vi "Test Runner Error Codes.vi"(8 "error in (no error)":errorcluster) -> (0 "error out":errorcluster)   [LabVIEW 2013]
uses:
  classes/Test Runner.Folder/Test Runner.Folder.lvclass
  classes/Test Runner/Test Runner.lvclass/Test Runner.ctl
  classes/Assert/Assert Equal Value_Variant.vi
  classes/Test/Test.lvclass
  classes/Assert/Assert.lvclass
  classes/Test Runner/Test Runner.lvclass
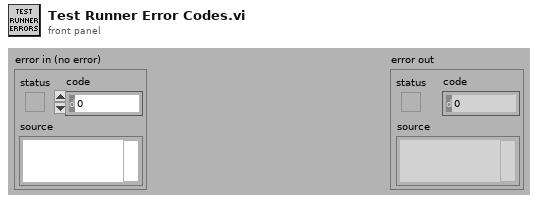
[diagram p1: front panel]
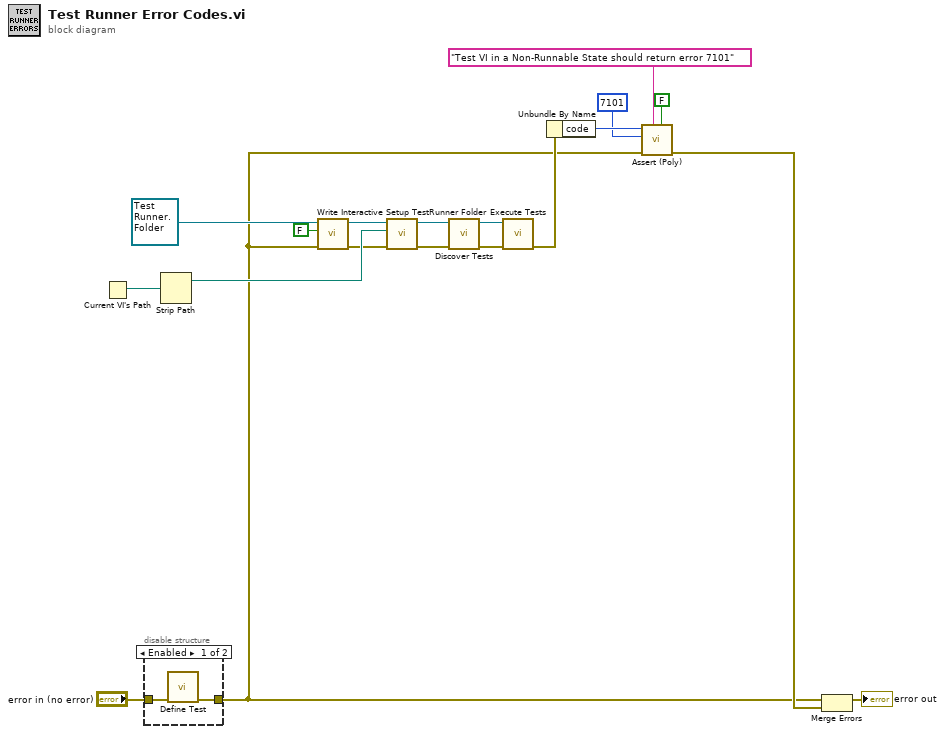
[diagram p0: block diagram]
diagram:
  n1 = Current VI's Path() -> (path=w7:path)
  n2 = disable-structure shown="Enabled" {
    disable-tunnel: "error in (no error)" -> [w20 w21]
    disable-tunnel: [w19 w21] -> w1
    frame Enabled {
      n3 = call "Define Test.vi"("error in (no error)"=w20) -> ("error out"=w19:errorcluster)  [unwired: 10 in]
    }
    frame Disabled {
    }
  }
  n4 = Strip Path(path=w7) -> (stripped path=w6:path)  [unwired: 1 out]
  n5 = call "Write Interactive.vi"("Interactive"=FALSE, "Test Runner in"=refnum<class "Test Runner.Folder.lvclass"> refnum ("Caraya.lvlib:Test Runner.Folder.lvclass")) -> ("Test Runner out"=w5:refnum<class "Test Runner.Folder.lvclass">)  [unwired: 9 in]
  n6 = call "Setup TestRunner Folder.vi"("error in (no error)"=w1, "Directory to search"=w6, "Test Runner.Folder"=w5) -> ("error out"=w8:errorcluster, "Test Runner.Folder out"=w12:refnum<class "Test Runner.Folder.lvclass">)  [unwired: 7 in]
  n7 = call "Discover Tests.vi"("error in (no error)"=w8, "Test Runner in"=w12) -> ("error out"=w11:errorcluster, "Test Runner out"=w9:refnum<class "Test Runner.Folder.lvclass">)  [unwired: 8 in]
  n8 = call-dynamic "Execute Tests.vi"("error in (no error)"=w11, "Test Runner in"=w9) -> ("error out"=w10:errorcluster)  [unwired: 8 in, 1 out]
  n9 = Unbundle By Name(w10) -> ("code"=w16:i32)
  n10 = call-poly "Assert (Poly).vi"("Assert Only? (F)"=FALSE, "Label"="Test VI in a Non-Runnable State should return error 7101", "error in (no error)"=w1, "Y"=7101 ("code"), "X"=w16) -> ("error out"=w13:errorcluster)  [unwired: 6 in]
  n11 = Merge Errors(w1, w13) -> (→"error out":errorcluster)
